vi "ConfigureMeasurementParameters.vi"(0 "Keysight_34401A-DMM in":refnum<class "Keysight_34401A-DMM.lvclass">, 5 "Configure_Parameters":variant, 11 "error in":errorcluster) -> (4 "Keysight_34401A-DMM out":refnum<class "Keysight_34401A-DMM.lvclass">, 15 "error out":errorcluster)   [LabVIEW 2020, in "Abstract_Instrument.lvlib" / "Keysight_34401A-DMM.lvclass"]
uses:
  Keysight_34401A-DMM.lvclass
  TypeDef/Configuration_Parameters.ctl
  <instrlib>/Agilent 34401/Agilent 34401.lvlib
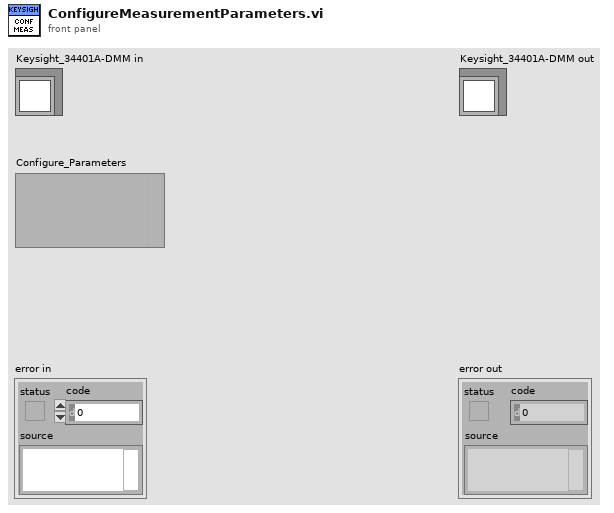
[diagram p1: front panel]
types:
  T1 = typedef "Abstract_Instrument.lvlib/Keysight_34401A-DMM.lvclass/Configuration_Parameters.ctl" = cluster{"Range":dbl, "Measurement Type":enum32{"DC Volts", "AC Volts", "DC Current", "AC Current", "2-wire Resistance", "4-wire Resistance", "Diode", "Frequency", "Period", "AC Volts DC Coupled", "Capacitance", "Inductance", "Temperature"}, "Resolution in Digits":enum32{"3 1/2", "4 1/2", "5 1/2", "6 1/2", "7 1/2"}, "pin or relay names":string[]}
  T2 = enum32{"3 1/2", "4 1/2", "5 1/2", "6 1/2", "7 1/2"}
  T3 = enum32{"DC Volts", "AC Volts", "DC Current", "AC Current", "2-wire Resistance", "4-wire Resistance", "Diode", "Frequency", "Period", "AC Volts DC Coupled", "Capacitance", "Inductance", "Temperature"}
  T4 = typedef "Abstract_Instrument.lvlib/Keysight_34401A-DMM.lvclass/Connection with Session.ctl" = cluster{"connection":T5, "session":refnum<visa-resource-name>}
  T5 = typedef "MeasurementLink Session Management V1.lvlib/Session Reservation.lvclass/Connection.ctl" = cluster{"pin or relay name":string, "site":i32, "instrument type id":string, "channel":string}
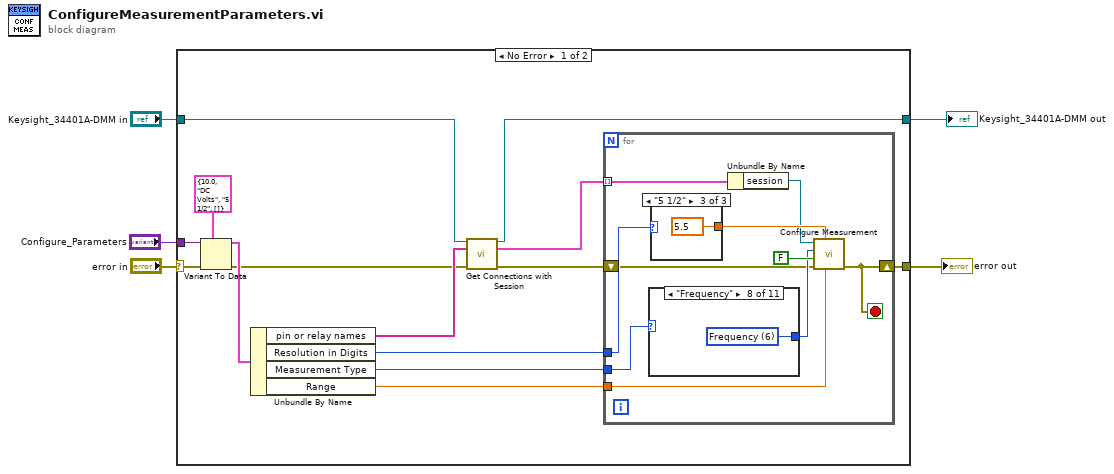
[diagram p0: block diagram]
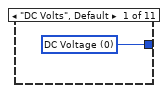
[diagram p2: hidden frame]
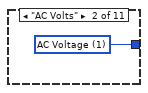
[diagram p3: hidden frame]
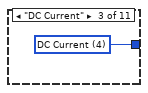
[diagram p4: hidden frame]
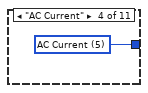
[diagram p5: hidden frame]
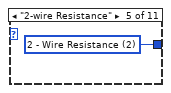
[diagram p6: hidden frame]
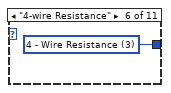
[diagram p7: hidden frame]
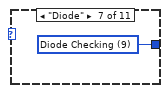
[diagram p8: hidden frame]
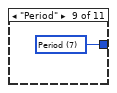
[diagram p9: hidden frame]
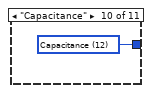
[diagram p10: hidden frame]
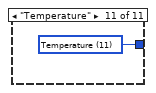
[diagram p11: hidden frame]
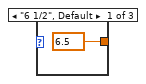
[diagram p12: hidden frame]
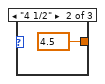
[diagram p13: hidden frame]
diagram:
  n1 = case shown="No Error" "error in" {
    selector: "error in" -> [w19 w44]
    tunnel: "Keysight_34401A-DMM in" -> [w10 w45]
    tunnel: "Configure_Parameters" -> [w18 _]
    tunnel: [w6 w45] -> w2
    tunnel: [w16 w44] -> w1
    frame No Error {
      n2 = Variant To Data(error in=w19, type=T1 {"Range"=10.0, "Measurement Type"=enum."DC Volts", "Resolution in Digits"=enum."5 1/2", "pin or relay names"=[]} ("Configure_Parameters"), Variant=w18) -> (data=w15:T1, error out=w9:errorcluster)
      n3 = Unbundle By Name(w15) -> ("pin or relay names"=w11:string[], "Resolution in Digits"=w13:T2, "Measurement Type"=w12:T3, "Range"=w14:dbl)
      n4 = call "Get Connections with Session.vi"("Keysight_34401A-DMM in"=w10, "pin or relay names"=w11, "error in (no error)"=w9) -> ("Keysight_34401A-DMM out"=w6:refnum<class "Keysight_34401A-DMM.lvclass">, "connections"=w7:T4[], "error out"=w8:errorcluster)  [unwired: 10 in]
      n5 = for {
        tunnel: w14 -> [w29]
        tunnel: w13 -> [w27]
        tunnel: w12 -> [w24]
        shift-right: [w20] -> w16
        shift-left: w8 -> [w23]
        tunnel: w7 -> [w21] mode=indexing
        stop <- w20 stop-if-true
        n6 = case shown="\"Frequency\"" w24 {
          tunnel: [w30 w31 w32 w33 w34 w35 w36 w37 w38 w39 w40] -> w25
          frame "DC Volts", Default {
            w30 = u16 0 items=["DC Voltage", "AC Voltage", "2 - Wire Resistance", "4 - Wire Resistance", "DC Current", "AC Current", "Frequency", "Period", "Continuity", "Diode Checking", "VDC:VDC Ratio", "Temperature", "Capacitance"] ("Function (0: DC Voltage)")
          }
          frame "AC Volts" {
            w31 = u16 1 items=["DC Voltage", "AC Voltage", "2 - Wire Resistance", "4 - Wire Resistance", "DC Current", "AC Current", "Frequency", "Period", "Continuity", "Diode Checking", "VDC:VDC Ratio", "Temperature", "Capacitance"] ("Function (0: DC Voltage)")
          }
          frame "DC Current" {
            w32 = u16 4 items=["DC Voltage", "AC Voltage", "2 - Wire Resistance", "4 - Wire Resistance", "DC Current", "AC Current", "Frequency", "Period", "Continuity", "Diode Checking", "VDC:VDC Ratio", "Temperature", "Capacitance"] ("Function (0: DC Voltage)")
          }
          frame "AC Current" {
            w33 = u16 5 items=["DC Voltage", "AC Voltage", "2 - Wire Resistance", "4 - Wire Resistance", "DC Current", "AC Current", "Frequency", "Period", "Continuity", "Diode Checking", "VDC:VDC Ratio", "Temperature", "Capacitance"] ("Function (0: DC Voltage)")
          }
          frame "2-wire Resistance" {
            w34 = u16 2 items=["DC Voltage", "AC Voltage", "2 - Wire Resistance", "4 - Wire Resistance", "DC Current", "AC Current", "Frequency", "Period", "Continuity", "Diode Checking", "VDC:VDC Ratio", "Temperature", "Capacitance"] ("Function (0: DC Voltage)")
          }
          frame "4-wire Resistance" {
            w35 = u16 3 items=["DC Voltage", "AC Voltage", "2 - Wire Resistance", "4 - Wire Resistance", "DC Current", "AC Current", "Frequency", "Period", "Continuity", "Diode Checking", "VDC:VDC Ratio", "Temperature", "Capacitance"] ("Function (0: DC Voltage)")
          }
          frame "Diode" {
            w36 = u16 9 items=["DC Voltage", "AC Voltage", "2 - Wire Resistance", "4 - Wire Resistance", "DC Current", "AC Current", "Frequency", "Period", "Continuity", "Diode Checking", "VDC:VDC Ratio", "Temperature", "Capacitance"] ("Function (0: DC Voltage)")
          }
          frame "Frequency" {
            w37 = u16 6 items=["DC Voltage", "AC Voltage", "2 - Wire Resistance", "4 - Wire Resistance", "DC Current", "AC Current", "Frequency", "Period", "Continuity", "Diode Checking", "VDC:VDC Ratio", "Temperature", "Capacitance"] ("Function (0: DC Voltage)")
          }
          frame "Period" {
            w38 = u16 7 items=["DC Voltage", "AC Voltage", "2 - Wire Resistance", "4 - Wire Resistance", "DC Current", "AC Current", "Frequency", "Period", "Continuity", "Diode Checking", "VDC:VDC Ratio", "Temperature", "Capacitance"] ("Function (0: DC Voltage)")
          }
          frame "Capacitance" {
            w39 = u16 12 items=["DC Voltage", "AC Voltage", "2 - Wire Resistance", "4 - Wire Resistance", "DC Current", "AC Current", "Frequency", "Period", "Continuity", "Diode Checking", "VDC:VDC Ratio", "Temperature", "Capacitance"] ("Function (0: DC Voltage)")
          }
          frame "Temperature" {
            w40 = u16 11 items=["DC Voltage", "AC Voltage", "2 - Wire Resistance", "4 - Wire Resistance", "DC Current", "AC Current", "Frequency", "Period", "Continuity", "Diode Checking", "VDC:VDC Ratio", "Temperature", "Capacitance"] ("Function (0: DC Voltage)")
          }
        }
        n7 = case shown="\"5 1/2\"" w27 {
          tunnel: [w41 w42 w43] -> w28
          frame "6 1/2", Default {
            w41 = 6.5 items=["4.5"=4.5, "5.5"=5.5, "6.5"=6.5] ("Manual Resolution (5.5 Digits)")
          }
          frame "4 1/2" {
            w42 = 4.5 items=["4.5"=4.5, "5.5"=5.5, "6.5"=6.5] ("Manual Resolution (5.5 Digits)")
          }
          frame "5 1/2" {
            w43 = 5.5 items=["4.5"=4.5, "5.5"=5.5, "6.5"=6.5] ("Manual Resolution (5.5 Digits)")
          }
        }
        n8 = Unbundle By Name(w21) -> ("session"=w22:refnum<visa-resource-name>)
        n9 = call <instrlib>:"Configure Measurement.vi"("Manual Range (1.00)"=w29, "Manual Resolution (5.5 Digits)"=w28, "error in (no error)"=w23, "Enable Auto Range (T: Enable)"=FALSE, "Function (0: DC Voltage)"=w25, "VISA resource name"=w22) -> ("error out"=w20:errorcluster)  [unwired: 4 in, 1 out]
      }
    }
    frame Error {
    }
  }
  "error out" <- w1
  "Keysight_34401A-DMM out" <- w2
